vi "SetTemperature.vi"(8 "error in (no error)":errorcluster, 10 "Temperature(degC)":dbl, 11 "Photometrics Cam v2 in":refnum<class "Photometrics_CH-250_Cam.lvclass">) -> (0 "error out":errorcluster, 2 "Success?":bool, 3 "Photometrics Cam v2 out":refnum<class "Photometrics_CH-250_Cam.lvclass">)   [LabVIEW 2013, in "Photometrics_CH-250_Cam.lvclass"]
doc: "Set and verify the camera TEMP_SETPOINT"
uses:
  Photometrics_CH-250_Cam.lvclass
  CameraSessionClass/CS250-CameraHardwareClass.lvclass
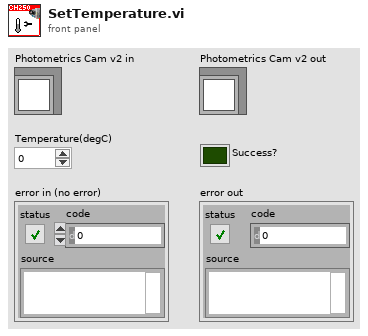
[diagram p1: front panel]
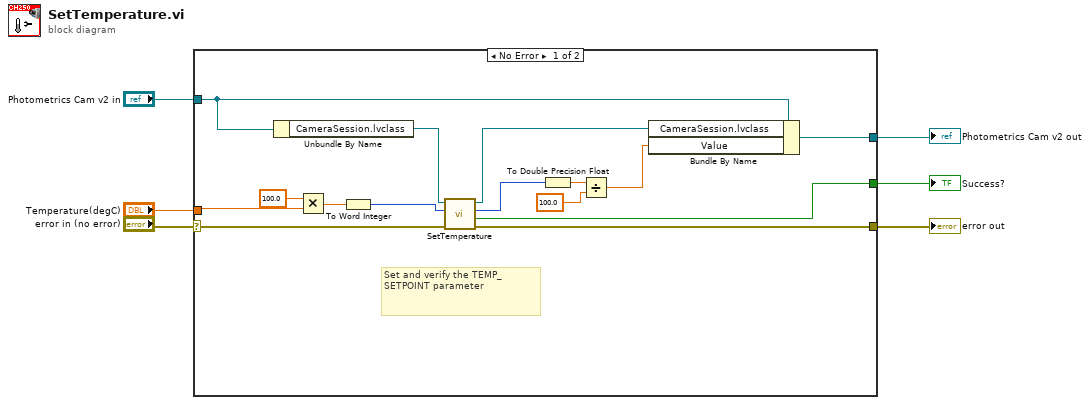
[diagram p0: block diagram]
diagram:
  n1 = case shown="No Error" "error in (no error)" {
    selector: "error in (no error)" -> [w16 w23]
    tunnel: [w21 w23] -> w6
    tunnel: "Temperature(degC)" -> [w15 _]
    tunnel: "Photometrics Cam v2 in" -> [w18 w22]
    tunnel: [w17 w22] -> w1
    tunnel: [w11 _] -> w2
    frame No Error {
      # "Set and verify the TEMP_SETPOINT parameter"
      n2 = Unbundle By Name(w18) -> ("CameraSession.lvclass"=w19:refnum<class "CS250-CameraHardwareClass.lvclass">)
      n3 = Multiply(x=100.0, y=w15) -> (x*y=w13:dbl)
      n4 = To Word Integer(number=w13) -> (16bit integer=w12:i16)
      n5 = call-dynamic "SetTemperature.vi"("error in (no error)"=w16, "TSetpoint(degC/100)"=w12, "CameraSession  in"=w19) -> ("error out"=w21:errorcluster, "Success"=w11:bool, "TSetpointReadback(degC/100)"=w10:i16, "CameraSession out"=w20:refnum<class "CS250-CameraHardwareClass.lvclass">)  [unwired: 5 in]
      n6 = To Double Precision Float(number=w10) -> (double precision float=w8:dbl)
      n7 = Divide(x=w8, y=100.0) -> (x/y=w7:dbl)
      n8 = Bundle By Name(cluster=w18, "CameraSession.lvclass"=w20, "Value"=w7) -> (w17:refnum<class "Photometrics_CH-250_Cam.lvclass">)
    }
    frame Error {
    }
  }
  "error out" <- w6
  "Photometrics Cam v2 out" <- w1
  "Success?" <- w2
